vi "HS_ReadWritePython.vi"(6 "Reply length":i32=-1, 7 "Timeouts (ms)":T1, 8 "error in":errorcluster, 9 "Console In":string, 10 "Write":string, 11 "VISA in":refnum<visa-resource-name>) -> (0 "error out":errorcluster, 1 "Console Out":string, 2 "Update?":bool, 3 "VISA out":refnum<visa-resource-name>, 4 "Not Done?":bool, 5 "read buffer":string)   [LabVIEW 2016]
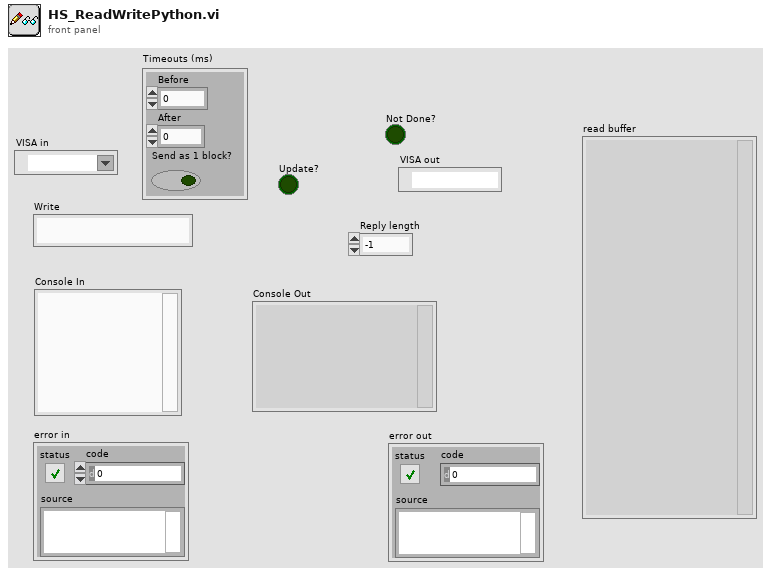
[diagram p1: front panel]
types:
  T1 = cluster{"Before":u8, "After":u8, "Send as 1 block?":bool}
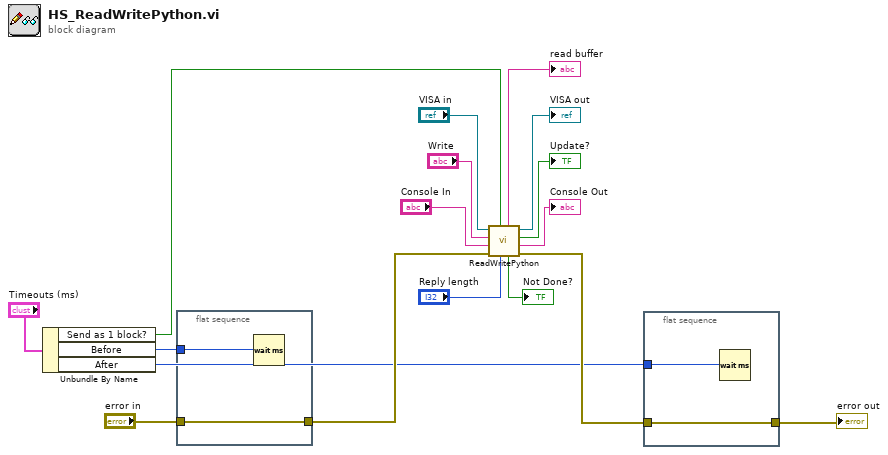
[diagram p0: block diagram]
diagram:
  n1 = Unbundle By Name("Timeouts (ms)") -> ("Send as 1 block?"=w1:bool, "Before"=w5:u8, "After"=w2:u8)
  n2 = flat-sequence {
    tunnel: [w19] -> w8
    tunnel: "error in" -> [w19]
    tunnel: w5 -> [w18]
    frame #0 {
      n3 = Wait (ms)(milliseconds to wait=w18) -> ()  [unwired: 1 out]
    }
  }
  n4 = call "ReadWritePython.vi"("Reply length"="Reply length", "Send as 1 block?"=w1, "error in"=w8, "Console In"="Console In", "Write"="Write", "VISA in"="VISA in") -> ("error out"=w4:errorcluster, "Console Out"=→"Console Out":string, "Update?"=→"Update?":bool, "VISA out"=→"VISA out":refnum<visa-resource-name>, "Not Done?"=→"Not Done?":bool, "read buffer"=→"read buffer":string)
  n5 = flat-sequence {
    tunnel: [w21] -> w3
    tunnel: w4 -> [w21]
    tunnel: w2 -> [w20]
    frame #0 {
      n6 = Wait (ms)(milliseconds to wait=w20) -> ()  [unwired: 1 out]
    }
  }
  "error out" <- w3
